vi "Get Relay States.vi"(8 "error in (no error)":errorcluster, 9 "nodePath":string, 10 "NIVS.System Definition Root":refnum<k24>, 11 "WorkspaceManager in":T1) -> (0 "error out":errorcluster, 1 "MUX Name":string, 2 "Relays":T2[](array[typedef]), 3 "WorkspaceManager out":T1)   [LabVIEW 2013]
uses:
  NationalInstruments.VeriStand.SystemStorage
  SubVIs/Relay Data.ctl
  SubVIs/Switch.ctl
  <vilib>/NI Veristand/Execution/Workspace/WorkspaceAPI.ctl
  NationalInstruments.VeriStand.ClientAPI
  NationalInstruments.VeriStand
  <vilib>/NI Veristand/Execution/Workspace/NI VeriStand - Get Single Channel Value.vi
  MUX Custom Device.lvlib
  <vilib>/NI Veristand/Execution/Workspace/NI_VS Workspace ExecutionAPI.lvlib
  NationalInstruments.VeriStand.SystemDefinitionAPI
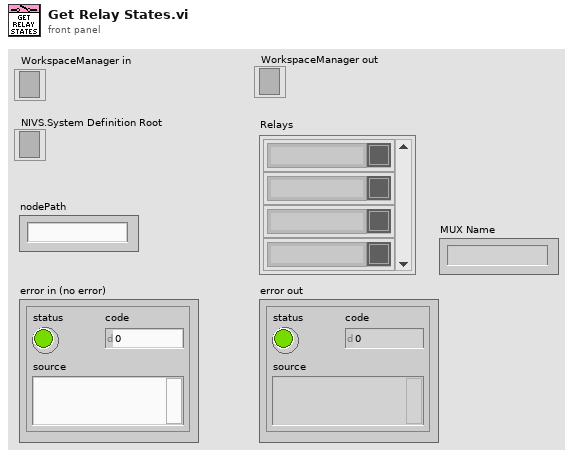
[diagram p1: front panel]
types:
  T1 = typedef "NI_VS Workspace ExecutionAPI.lvlib/WorkspaceAPI.ctl" = refnum<k24>
  T2 = typedef "MUX Custom Device.lvlib/Relay Data.ctl" = cluster{"Relay Name":string, "State":T3}
  T3 = typedef "MUX Custom Device.lvlib/Switch.ctl" = bool
  T4 = typedef "NI_VS Workspace ExecutionAPI.lvlib/SystemState.ctl" = u8
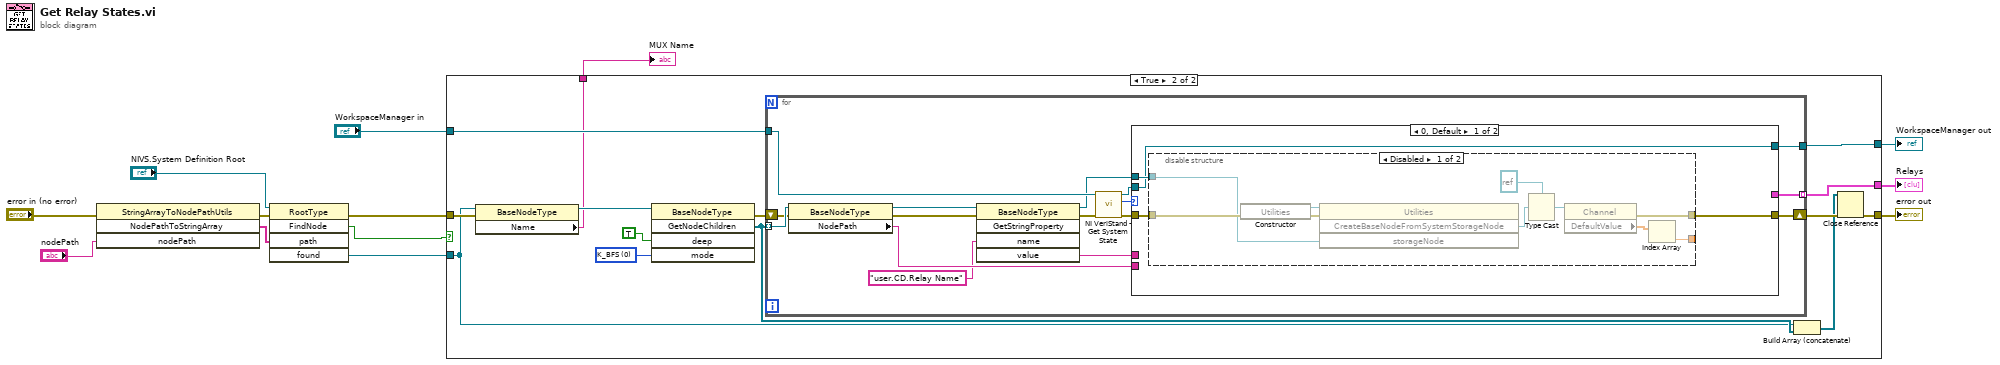
[diagram p0: block diagram]
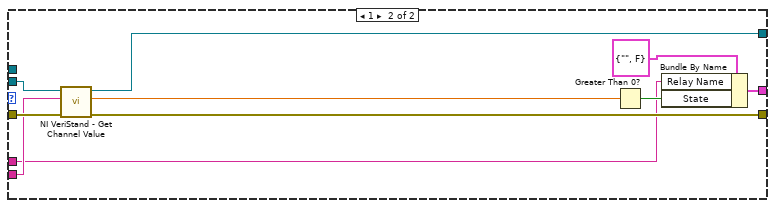
[diagram p4: hidden frame]
diagram:
  n1 = invoke class="StringArrayToNodePathUtils" method="NodePathToStringArray"(error in="error in (no error)", "nodePath"="nodePath") -> (error out=w12:errorcluster, "NodePathToStringArray"=w13:string[])  [unwired: 2 in, 2 out]
  n2 = invoke class="RootType" method="FindNode"(reference="NIVS.System Definition Root", error in=w12, "path"=w13) -> (error out=w2:errorcluster, "FindNode"=w9:bool, "found"=w8:refnum<k24>)  [unwired: 2 in, 2 out]
  n3 = case shown="True" w9 {
    tunnel: w2 -> [w15 w19]
    tunnel: w8 -> [_ w18]
    tunnel: "WorkspaceManager in" -> [w14 w26]
    tunnel: [w14 w25] -> w6
    tunnel: [w15 w22] -> w5
    tunnel: [_ w24] -> w4
    tunnel: [_ w16] -> w1
    frame False {
    }
    frame True {
      w28 = 0 items=["K_BFS", "K_DFS", "K_CHILDONLY", "K_UP"] ("mode")
      n4 = property class="BaseNodeType"(reference=w18, error in=w19) -> (reference out=w17:refnum<k24>, "Name"=w16:string)  [unwired: 1 out]
      n5 = invoke class="BaseNodeType" method="GetNodeChildren"(reference=w17, "deep"=TRUE, "mode"=w28) -> (error out=w27:errorcluster, "GetNodeChildren"=w21:refnum<k24>[])  [unwired: 2 in, 3 out]
      n6 = for {
        tunnel: w21 -> [w45] mode=indexing
        shift-right: [w42] -> w23
        shift-left: w27 -> [w44]
        tunnel: w26 -> [w41]
        tunnel: [w43] -> w25
        tunnel: [w30] -> w24 mode=indexing
        n7 = property class="BaseNodeType"(reference=w45, error in=w44) -> (reference out=w32:refnum<k24>, error out=w33:errorcluster, "NodePath"=w35:string)
        n8 = invoke class="BaseNodeType" method="GetStringProperty"(reference=w32, error in=w33, "name"="user.CD.Relay Name") -> (reference out=w36:refnum<k24>, error out=w40:errorcluster, "value"=w31:string)  [unwired: 2 in, 2 out]
        n9 = call <vilib>:"NI VeriStand - Get System State.vi"("error in (no error)"=w40, "WorkspaceManager in"=w41) -> ("error out"=w39:errorcluster, "System State"=w38:T4, "WorkspaceManager  out"=w37:T1)  [unwired: 5 in, 2 out]
        n10 = case shown="0, Default" w38 {
          tunnel: w39 -> [w49 w69]
          tunnel: w37 -> [w46 w68]
          tunnel: [w46 w67] -> w43
          tunnel: [w47 w66] -> w42
          tunnel: w35 -> [_ w65]
          tunnel: w36 -> [w48 _]
          tunnel: w31 -> [_ w61]
          tunnel: [_ w60] -> w30
          frame 0, Default {
            n11 = disable-structure shown="Disabled" {
              disable-tunnel: w49 -> [w54 _]
              disable-tunnel: w48 -> [w53 _]
              disable-tunnel: [w52 _] -> w47
              disable-tunnel: [w50 _] -> _
              frame Disabled {
                n12 = constructor class="Utilities"(error in=w54) -> (reference out=w55:refnum<k24>, error out=w56:errorcluster)  [unwired: 2 in, 1 out]
                n13 = invoke class="Utilities" method="CreateBaseNodeFromSystemStorageNode"(reference=w55, error in=w56, "storageNode"=w53) -> ("CreateBaseNodeFromSystemStorageNode"=w57:refnum<k24>)  [unwired: 1 in, 3 out]
                n14 = Type Cast(type=refnum<k24> refnum ("CreateBaseNodeFromSystemStorageNode"), x=w57) -> (*(type *) &x=w59:refnum<k24>)
                n15 = property class="Channel"(reference=w59) -> (error out=w52:errorcluster, "DefaultValue"=w51:dbl[])  [unwired: 1 in, 1 out]
                n16 = Index Array(array=w51) -> (element=w50:dbl)  [unwired: 1 in]
              }
              frame Enabled {
              }
            }
          }
          frame 1 {
            n17 = call-poly <vilib>:"NI VeriStand - Get Channel Value.vi"("error in (no error)"=w69, "Channel"=w65, "WorkspaceManager in"=w68) -> ("error out"=w66:errorcluster, "Value"=w62:dbl, "WorkspaceManager out"=w67:T1)  [unwired: 6 in]
            n18 = Greater Than 0?(x=w62) -> (x > 0?=w64:bool)
            n19 = Bundle By Name(cluster=T2 {"Relay Name"="", "State"=FALSE} ("Relay Data"), "Relay Name"=w61, "State"=w64) -> (w60:T2)
          }
        }
      }
      n20 = Build Array (concatenate)(w18, w21) -> (w20:refnum<k24>[])
      n21 = Close Reference(reference=w20, error in (no error)=w23) -> (error out=w22:errorcluster)
    }
  }
  "Relays" <- w4
  "WorkspaceManager out" <- w6
  "error out" <- w5
  "MUX Name" <- w1
